vi "construct.vi"(6 "tablecloth_type":T1 items=["Type 1", "Type 2"], 8 "error in (no error)":errorcluster, 9 "cost":dbl, 10 "id":u32) -> (0 "error out":errorcluster, 3 "table out":refnum<class "Table.lvclass">)   [LabVIEW 2021, in "Table.lvclass"]
uses:
  Table.lvclass
  ITable/TableclothType.ctl
  Table.lvclass/Table.ctl
  ITable/ITable.lvclass
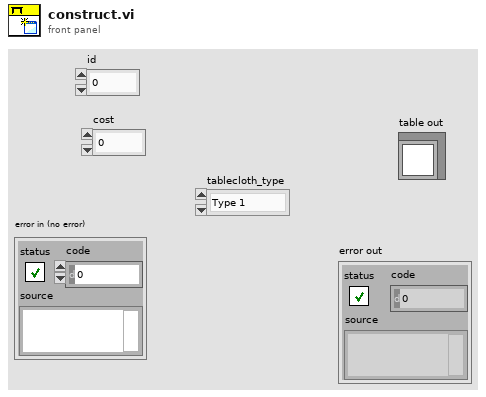
[diagram p1: front panel]
types:
  T1 = typedef "ITable.lvclass/TableclothType.ctl" = u16
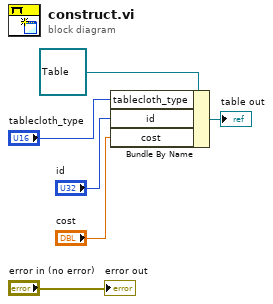
[diagram p0: block diagram]
diagram:
  n1 = Bundle By Name(cluster=refnum<class "Table.lvclass"> refnum ("Table.lvclass"), "tablecloth_type"="tablecloth_type", "id"="id", "cost"="cost") -> (→"table out":refnum<class "Table.lvclass">)
  "error out" <- "error in (no error)"
